vi "Array of Variants to JSON Object.vi"(4 "LVClass Serializer":refnum<class "JSONtext LVClass Serializer.lvclass">, 5 "enable LabVIEW extensions? (T)":bool=TRUE, 6 "Pretty Print?":bool, 9 "error in (no error)":errorcluster, 10 "Names":string[](array[string]), 11 "Array":variant[](array[variant])) -> (1 "error out":errorcluster, 3 "<JSON>":string caption="<JSON>Object")   [LabVIEW 2020, in "JSONtext.lvlib"]
doc: "Flatten an Array of Variants into a JSON Object. If item names are not supplied, they will be taken from the data name in the Variants.\n\nStrings or Arrays of strings marked with a leading <JSON> tag in their name (including inside clusters) are treated as already being valid JSON. Strings not marked as <JSON> are quoted and escaped as a JSON String."
uses:
  <vilib>/JDP Science/JSONtext/JSONtext.lvlib
  <vilib>/JDP Science/JSONtext/LVClass Serializer/JSONtext LVClass Serializer.lvclass
  <vilib>/Utility/Data Type/NI_Data Type.lvlib
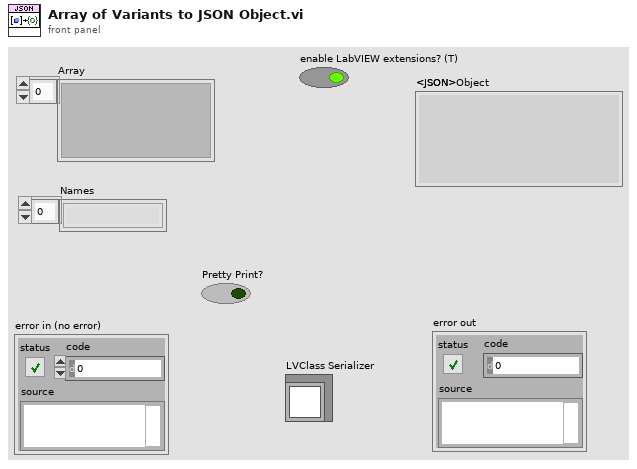
[diagram p1: front panel]
types:
  T1 = typedef "NI_Data Type.lvlib/Data Type.ctl" = enum8{"Invalid Type", "Void", "I8", "I16", "I32", "I64", "U8", "U16", "U32", "U64", "Single Float", "Double Float", "Extended Float", "Single Complex", "Double Complex", "Extended Complex", "Enum U8", "Enum U16", "Enum U32", "Enum U64", "Single Float With Unit", "Double Float With Unit", "Extended Float With Unit", "Single Complex with Unit", "Double Complex with Unit", "Extended Complex with Unit", "Boolean", "String", "Path", "Picture", "Tag", "Array", "Cluster", "Variant", "LV Variant", "Waveform", "Timestamp", "Digital Waveform", "Digital Data", "ExpressData", "Refnum", "External Data", "VI", "Poly VI", "LabVIEW Class Instance", "Fixed Point", "Set Collection", "Map Collection"}
  T2 = typedef "JSONtext.lvlib/Tag Type.ctl" = enum16{"No Tag", "<JSON>", "<JOBJ>"}
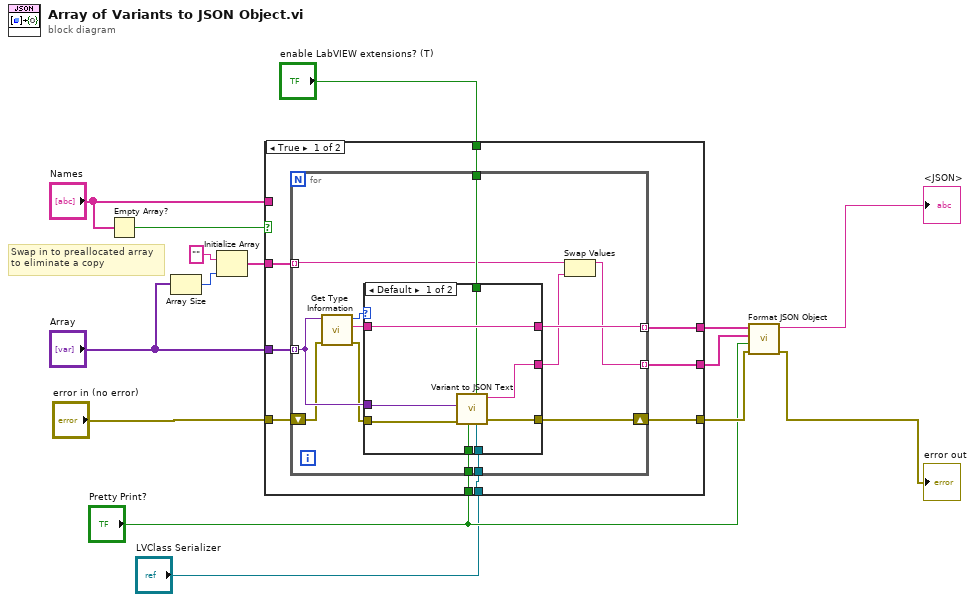
[diagram p0: block diagram]
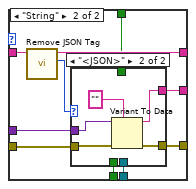
[diagram p2: hidden frame]
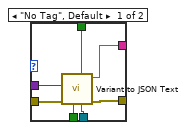
[diagram p3: hidden frame]
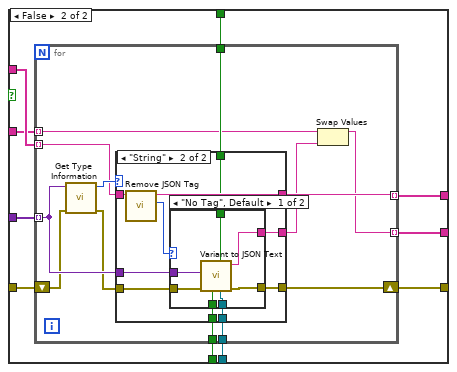
[diagram p4: hidden frame]
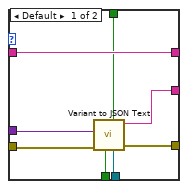
[diagram p5: hidden frame]
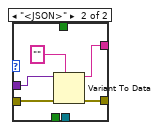
[diagram p6: hidden frame]
diagram:
  # "Swap in to preallocated array\nto eliminate a copy"
  n1 = Empty Array?(array="Names") -> (empty?=w9:bool)
  n2 = Array Size(array="Array") -> (size(s)=w2:i32)
  n3 = Initialize Array("", w2) -> (w1:string[])
  n4 = case shown="True" w9 {
    tunnel: [w24 w77] -> w14
    tunnel: [w23 w76] -> w12
    tunnel: [w22 w75] -> w11
    tunnel: "error in (no error)" -> [w21 w74]
    tunnel: "Array" -> [w20 w73]
    tunnel: "Names" -> [_ w70]
    tunnel: "Pretty Print?" -> [w19 w72]
    tunnel: "enable LabVIEW extensions? (T)" -> [w18 w71]
    tunnel: "LVClass Serializer" -> [w17 w69]
    tunnel: w1 -> [w16 w68]
    frame True {
      n5 = for {
        shift-right: [w35] -> w24
        shift-left: w21 -> [w30]
        tunnel: w20 -> [w37] mode=indexing
        tunnel: [w26] -> w23 mode=indexing
        tunnel: [w34] -> w22 mode=indexing
        tunnel: w19 -> [w33]
        tunnel: w18 -> [w32]
        tunnel: w17 -> [w28]
        tunnel: w16 -> [w27] mode=indexing
        n6 = call <vilib>:"Get Type Information.vi"("error in (no error)"=w30, "variant"=w37) -> ("error out"=w29:errorcluster, "name"=w36:string, "type"=w31:T1)  [unwired: 5 in, 2 out]
        n7 = case shown="Default" w31 {
          tunnel: w37 -> [w40 w55]
          tunnel: w36 -> [w45 w54]
          tunnel: w29 -> [w41 w53]
          tunnel: [w44 w52] -> w35
          tunnel: [w45 w51] -> w34
          tunnel: w33 -> [w42 w50]
          tunnel: w32 -> [w43 w49]
          tunnel: [w39 w48] -> w25
          tunnel: w28 -> [w38 w46]
          frame Default {
            n8 = call <vilib>:"Variant to JSON Text.vi"("LVClass Serializer"=w38, "enable LabVIEW extensions? (T)"=w43, "Pretty Print?"=w42, "error in (no error)"=w41, "Variant"=w40) -> ("error out"=w44:errorcluster, "<JSON>"=w39:string)  [unwired: 4 in, 1 out]
          }
          frame "String" {
            n9 = call <vilib>:"Remove JSON Tag.vi"("Name"=w54) -> ("Tag"=w47:T2, "Name (tag stripped)"=w51:string)  [unwired: 9 in]
            n10 = case shown="\"<JSON>\"" w47 {
              tunnel: w55 -> [w62 w65]
              tunnel: w53 -> [w61 w66]
              tunnel: [w60 w67] -> w52
              tunnel: w50 -> [w59 _]
              tunnel: w49 -> [w58 _]
              tunnel: [w57 w63] -> w48
              tunnel: w46 -> [w56 _]
              frame "No Tag", Default {
                n11 = call <vilib>:"Variant to JSON Text.vi"("LVClass Serializer"=w56, "enable LabVIEW extensions? (T)"=w58, "Pretty Print?"=w59, "error in (no error)"=w61, "Variant"=w62) -> ("error out"=w60:errorcluster, "<JSON>"=w57:string)  [unwired: 4 in, 1 out]
              }
              frame "<JSON>" {
                n12 = Variant To Data(error in=w66, type="", Variant=w65) -> (data=w63:string, error out=w67:errorcluster)
              }
            }
          }
        }
        n13 = Swap Values(12:w27, 14:w25) -> (1:w26:string)  [unwired: 1 in, 1 out]
      }
    }
    frame False {
      n14 = for {
        shift-right: [w89] -> w77
        shift-left: w74 -> [w84]
        tunnel: w73 -> [w90] mode=indexing
        tunnel: [w79] -> w76 mode=indexing
        tunnel: [w88] -> w75 mode=indexing
        tunnel: w72 -> [w87]
        tunnel: w71 -> [w86]
        tunnel: w70 -> [w82] mode=indexing
        tunnel: w69 -> [w81]
        tunnel: w68 -> [w80] mode=indexing
        n15 = call <vilib>:"Get Type Information.vi"("error in (no error)"=w84, "variant"=w90) -> ("error out"=w83:errorcluster, "type"=w85:T1)  [unwired: 5 in, 3 out]
        n16 = case shown="\"String\"" w85 {
          tunnel: w90 -> [w93 w108]
          tunnel: w82 -> [w98 w107]
          tunnel: w83 -> [w94 w106]
          tunnel: [w97 w105] -> w89
          tunnel: [w98 w104] -> w88
          tunnel: w87 -> [w95 w103]
          tunnel: w86 -> [w96 w102]
          tunnel: [w92 w101] -> w78
          tunnel: w81 -> [w91 w99]
          frame Default {
            n17 = call <vilib>:"Variant to JSON Text.vi"("LVClass Serializer"=w91, "enable LabVIEW extensions? (T)"=w96, "Pretty Print?"=w95, "error in (no error)"=w94, "Variant"=w93) -> ("error out"=w97:errorcluster, "<JSON>"=w92:string)  [unwired: 4 in, 1 out]
          }
          frame "String" {
            n18 = call <vilib>:"Remove JSON Tag.vi"("Name"=w107) -> ("Tag"=w100:T2, "Name (tag stripped)"=w104:string)  [unwired: 9 in]
            n19 = case shown="\"No Tag\", Default" w100 {
              tunnel: w108 -> [w115 w118]
              tunnel: w106 -> [w114 w119]
              tunnel: [w113 w120] -> w105
              tunnel: w103 -> [w112 _]
              tunnel: w102 -> [w111 _]
              tunnel: [w110 w116] -> w101
              tunnel: w99 -> [w109 _]
              frame "No Tag", Default {
                n20 = call <vilib>:"Variant to JSON Text.vi"("LVClass Serializer"=w109, "enable LabVIEW extensions? (T)"=w111, "Pretty Print?"=w112, "error in (no error)"=w114, "Variant"=w115) -> ("error out"=w113:errorcluster, "<JSON>"=w110:string)  [unwired: 4 in, 1 out]
              }
              frame "<JSON>" {
                n21 = Variant To Data(error in=w119, type="", Variant=w118) -> (data=w116:string, error out=w120:errorcluster)
              }
            }
          }
        }
        n22 = Swap Values(12:w80, 14:w78) -> (1:w79:string)  [unwired: 1 in, 1 out]
      }
    }
  }
  n23 = call <vilib>:"Format JSON Object.vi"("error in (no error)"=w14, "Pretty Print?"="Pretty Print?", "JSON elements"=w12, "Names"=w11) -> ("error out"=→"error out":errorcluster, "JSON Object Text out"=→"<JSON>":string)  [unwired: 6 in]
